vi "ProbeStationAutomation.vi"() -> ()   [LabVIEW 2020]
uses:
  Control 2.ctl
  D:/LabviewDXFViewer/LabviewDXFViewer/bin/Release/LabviewDXFViewer.exe
  LabviewDXFViewer/bin/Release/LabviewDXFViewer.exe
  UIReferences.ctl
  WaferAlignmentType.ctl
  <vilib>/Utility/file.llb/Write Delimited Spreadsheet (DBL).vi
  Keithley 2600 Series/Keithley 2600 Series.lvlib
panel:
  in  "StartOxide":refnum<k24>(container)
  out "WaferAlignment":T1
  out "UiDefinition 3":T2
  in  "PathInfos":T3
  in  "UiDefinition 2":T2
  out "SweepInfo":T4
  out "error out":errorcluster
  out "Position 3":i32[](array[numeric])
  out "Position 2":i32[](array[numeric])
  out "Status":string="Please Load/Select probe site list"
  in  "Chip Orientation":i32(ring) items=["Horizontal", "Vertical"]
  in  "TextEditor":refnum<k24>(container)
  out "WaferTestPoints":string
  out "TestPointsLoaded":bool
  out "dxfFile":string
  out "error out 5":errorcluster
  out "Fit Array":string[][](array[string])
  out "error out 4":errorcluster
  out "error out 3":errorcluster
  out "Fit":dbl[][](array[numeric])
  out "IV Scan Data":dbl[][](array[numeric])
  out "Rotation Misalign":dbl[](array[numeric])
  out "Scale Misalign":dbl
  out "Position 1":i32[](array[numeric])
  in  "Microsites":refnum<k24>(container)
  in  "DXFCanvas":refnum<k24>(container)
  in  "WebCamViewer":refnum<k24>(container)
  in  "IV Curves":T5
  in  "Tab Control":T6(tab)
  in  "ClearPositions":bool
  in  "User":string
  in  "resetcontact":bool
  in  "EnableJoystick":bool
  in  "StartCycle":refnum<k24>(container)
  in  "Version":string
  in  "Experiment":string
  in  "Lower":refnum<k24>(container)
  in  "Raise":refnum<k24>(container)
  in  "West":refnum<k24>(container)
  in  "East":refnum<k24>(container)
  in  "North":refnum<k24>(container)
  in  "South":refnum<k24>(container)
  in  "Align Position 1":bool
  in  "Platten Move":refnum<k24>(container)
  in  "Masks":string(combo)
  in  "Move Position 1":bool
  in  "Align Position 3":bool
  in  "Position 3":bool
  in  "Align Position 2":bool
  in  "Position 2":bool
  in  "Die":string
  in  "Wafer":string
  in  "Jog (um) 2":dbl=100.0
  in  "Jog (um)":dbl=500.0
  in  "Load Mask":bool
  in  "Save Wafer":bool
  in  "Lift Distance (um)":dbl=2000.0
  in  "Quit":bool
  out "In Contact":bool
  out "Motor Position":string
  in  "Save Tag":string
  out "Capacitance":dbl
  in  "Current Range (A)":dbl=1e-10
  in  "Junction":string(combo)="None"
  in  "Sweeps":dbl=2.0
  in  "Number Points":dbl=200.0
  in  "Minimum (mV)":dbl=-100.0
  in  "Maxiumum (mV)":dbl=100.0
  in  "Source Measure Unit Channel (0: Channel A)":i32(ring) items=["Channel A", "Channel B"]
  in  "VISA resource name":refnum<visa-resource-name>="Keithley_2636A"
  in  "Scan":bool
  in  "Save Scan":bool
  out "Conductance":dbl
  out "Intercept":dbl
  out "XY Graph":cluster{"x":timestamp, "y":dbl}[](graph)
  in  "Steps Per micron":dbl=0.629
  in  "Stepper Controller Port":i32=3
  out "GetCameras":string[](array[string])
  in  "Wafer Definition File":path=path "C:/Users/User/Desktop/Automation/ASU FG Mask 21.08.26.dxf"
  in  "Wafer Units to microns":dbl=1.0
  in  "Data Path":path=path "C:/Users/User/Desktop/Automation/data"
  # "Run Oxide"
  # "Optional Tags"
  # "Jog Platten"
  # "Platten Altitude"
  # "Run IVs"
  # "Cycle Step"
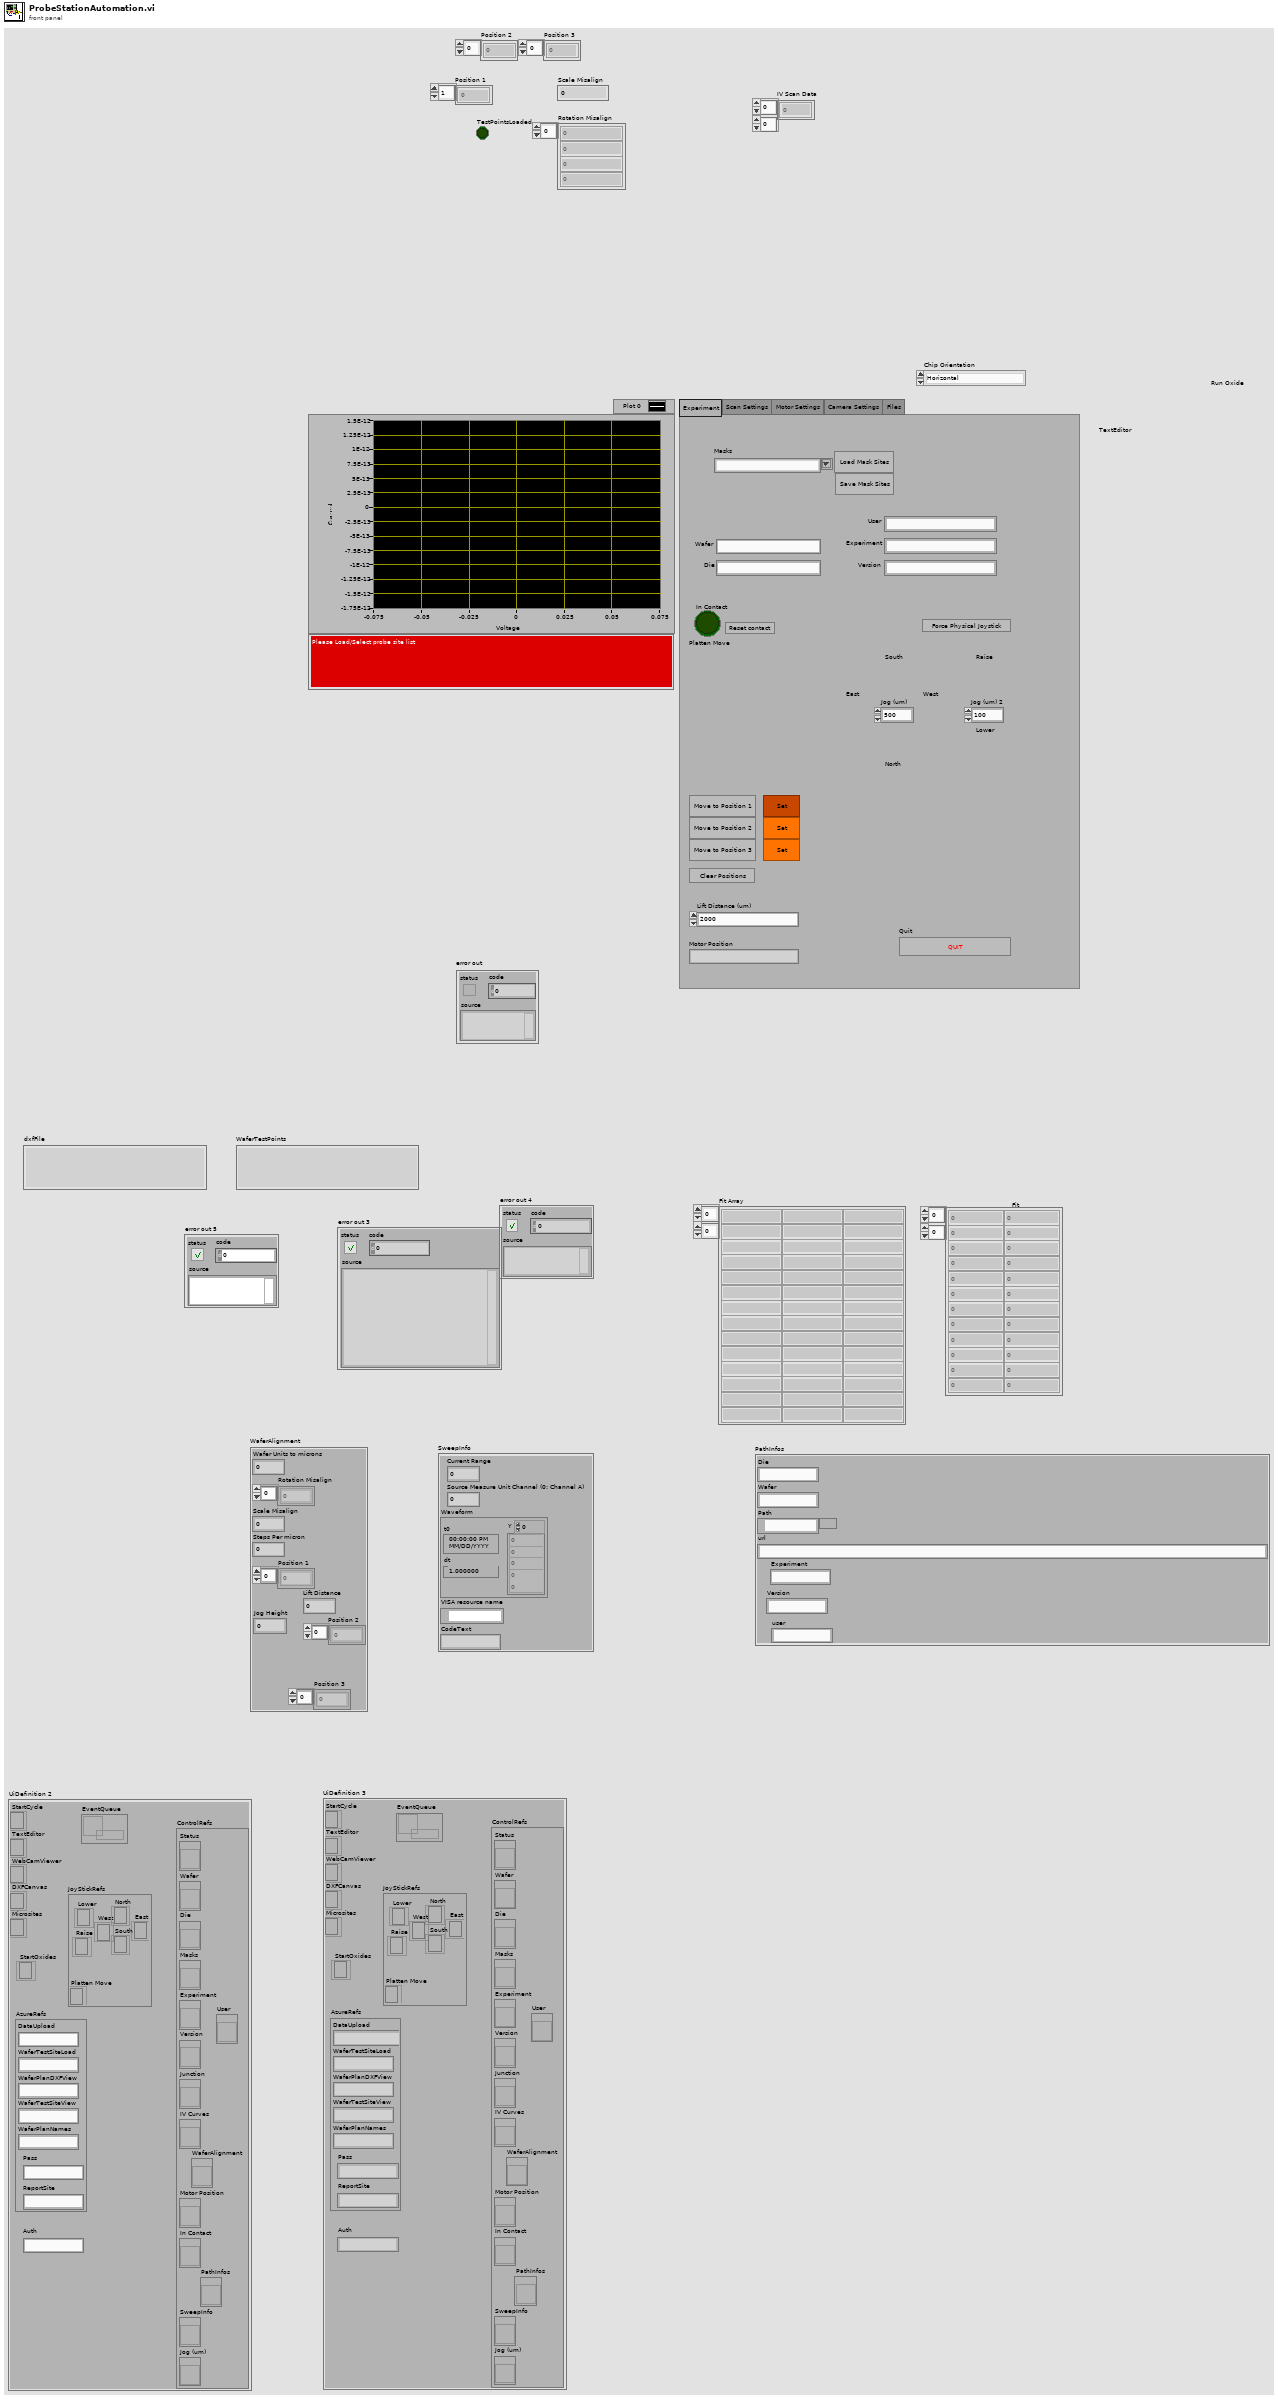
[diagram p1: front panel]
types:
  T1 = typedef "WaferAlignmentType.ctl" = cluster{"Wafer Units to microns":dbl, "Rotation Misalign":dbl[], "Scale Misalign":dbl, "Steps Per micron":dbl, "Position 1":i32[], "Position 2":i32[], "Lift Distance":i32, "Position 3":i32[], "Jog Height":i32}
  T2 = typedef "UIReferences.ctl" = cluster{"StartCycle":refnum<k24>, "TextEditor":refnum<k24>, "WebCamViewer":refnum<k24>, "DXFCanvas":refnum<k24>, "Microsites":refnum<k24>, "JoyStickRefs":cluster{"North":refnum<k24>, "Lower":refnum<k24>, "Raise":refnum<k24>, "Platten Move":refnum<k24>, "West":refnum<k24>, "East":refnum<k24>, "South":refnum<k24>}, "AzureRefs":cluster{"DataUpload":string, "WaferTestSiteLoad":string, "WaferPlanDXFView":string, "WaferTestSiteView":string, "WaferPlanNames":string, "Pass":string, "ReportSite":string}, "ControlRefs":cluster{"Status":refnum<vi>, "Wafer":refnum<vi>, "Die":refnum<vi>, "Masks":refnum<vi>, "Experiment":refnum<vi>, "Version":refnum<vi>, "Junction":refnum<vi>, "IV Curves":refnum<vi>, "Motor Position":refnum<vi>, "In Contact":refnum<vi>, "SweepInfo":refnum<vi>, "Jog (um)":refnum<vi>, "PathInfos":refnum<vi>, "User":refnum<vi>, "WaferAlignment":refnum<vi>}, "EventQueue":refnum<queue>, "StartOxides":refnum<k24>, "Auth":string}
  T3 = cluster{"Die":string, "Wafer":string, "Path":path, "url":string, "Experiment":string, "Version":string, "user":string}
  T4 = cluster{"Current Range":dbl, "Source Measure Unit Channel (0: Channel A)":i32, "Waveform":waveform(dbl), "VISA resource name":refnum<visa-resource-name>, "CodeText":string}
  T5 = typedef "Control 2.ctl" = cluster{"Y":dbl[], "Current (A)":dbl[]}
  T6 = enum32{"Experiment", "Scan Settings", "Motor Settings", "Camera Settings", "Files"}
  T7 = cluster{"DataUpload":string, "WaferTestSiteLoad":string, "WaferPlanDXFView":string, "WaferTestSiteView":string, "WaferPlanNames":string, "Pass":string, "ReportSite":string}
  T8 = cluster{"North":refnum<k24>, "Lower":refnum<k24>, "Raise":refnum<k24>, "Platten Move":refnum<k24>, "West":refnum<k24>, "East":refnum<k24>, "South":refnum<k24>}
  T9 = cluster{"Status":refnum<vi>, "Wafer":refnum<vi>, "Die":refnum<vi>, "Masks":refnum<vi>, "Experiment":refnum<vi>, "Version":refnum<vi>, "Junction":refnum<vi>, "IV Curves":refnum<vi>, "Motor Position":refnum<vi>, "In Contact":refnum<vi>, "SweepInfo":refnum<vi>, "Jog (um)":refnum<vi>, "PathInfos":refnum<vi>, "User":refnum<vi>, "WaferAlignment":refnum<vi>}
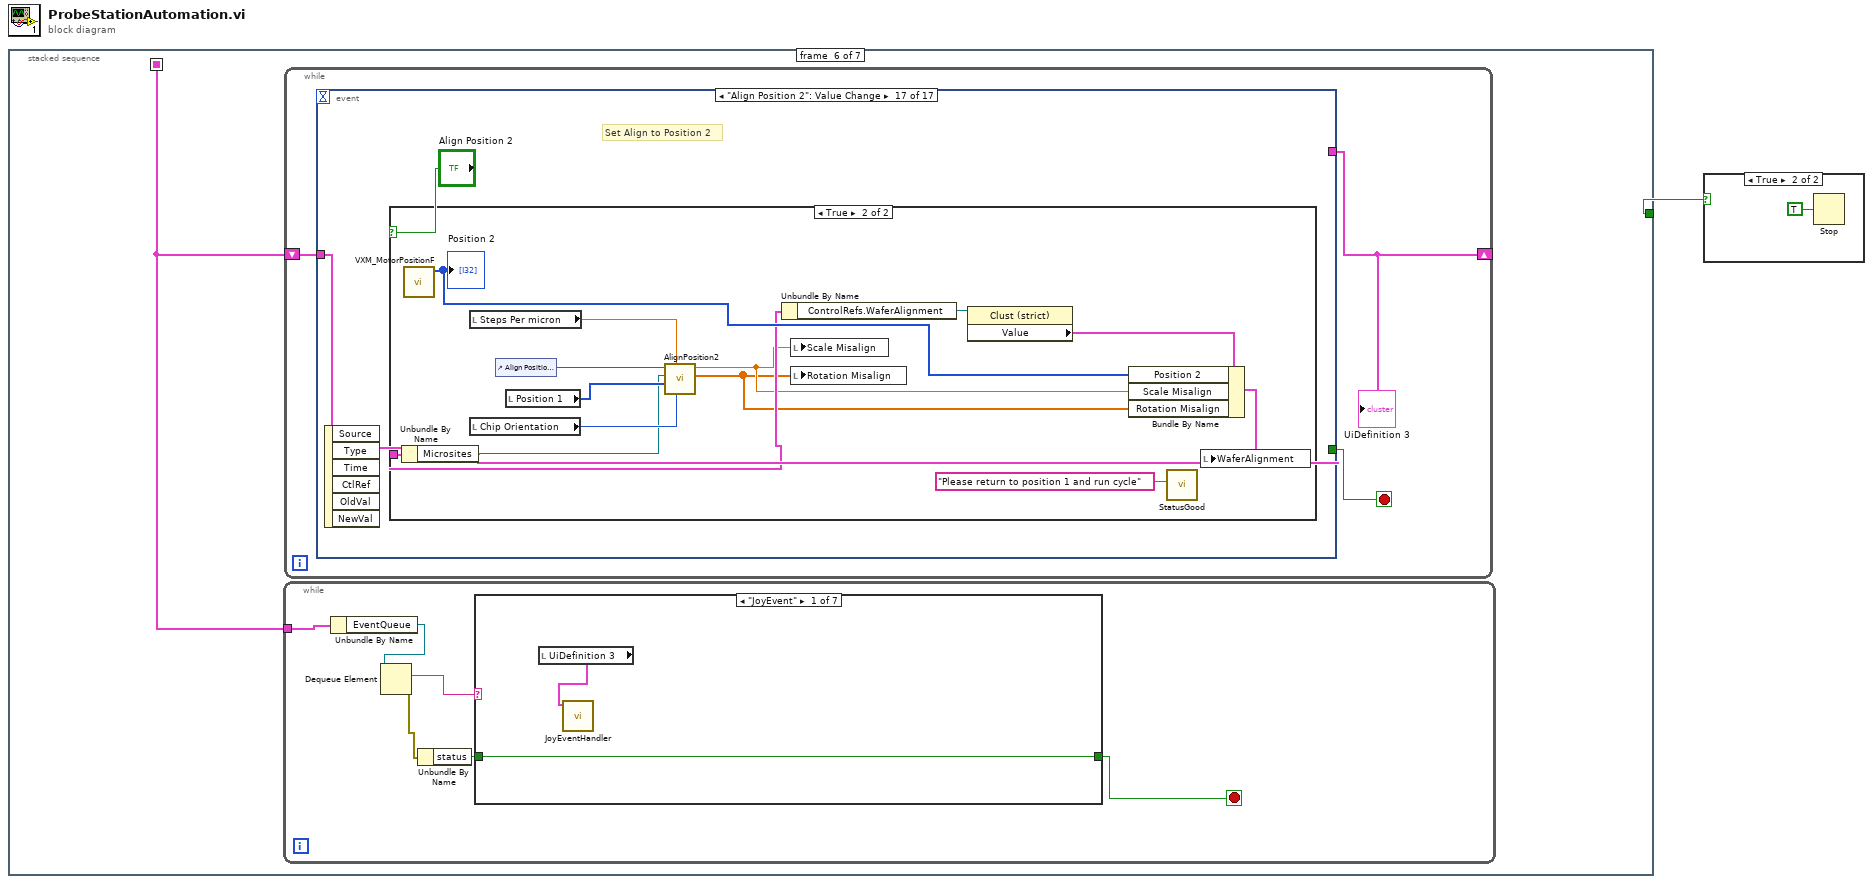
[diagram p0: block diagram]
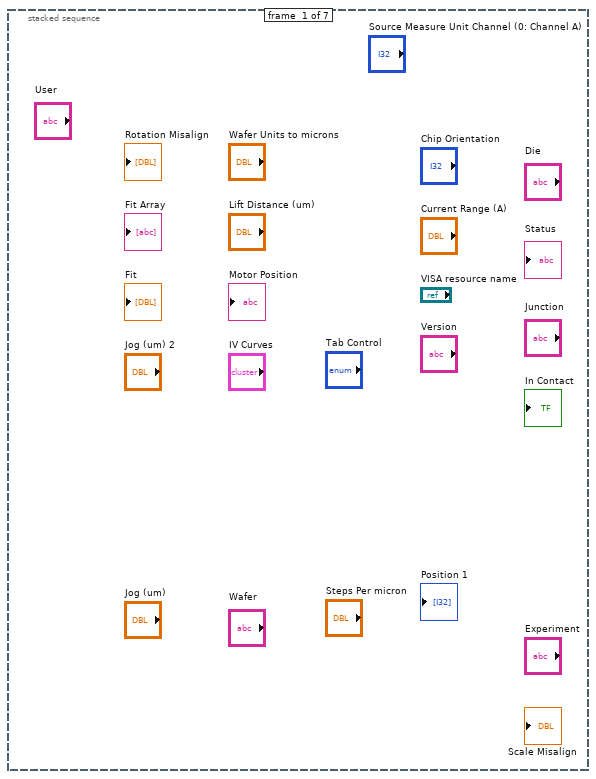
[diagram p3: hidden frame]
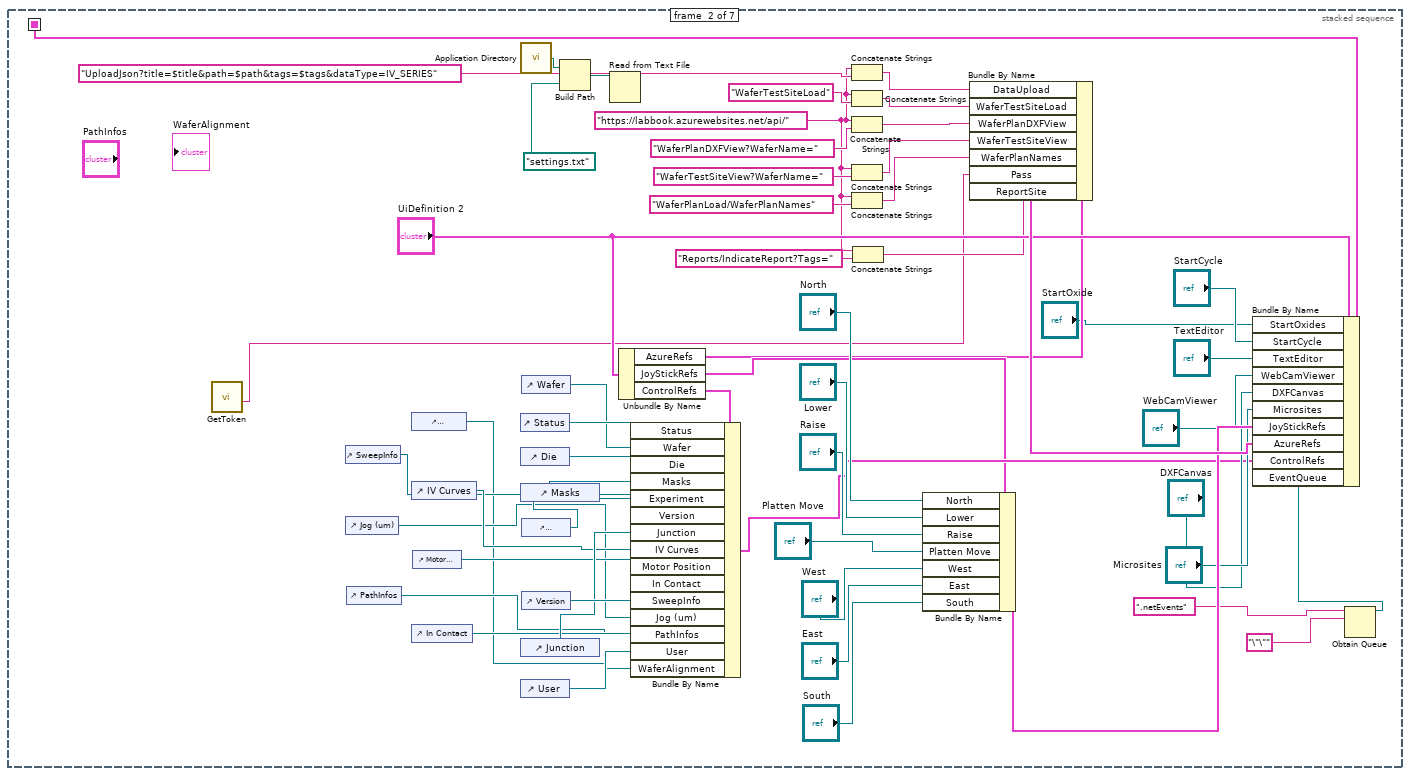
[diagram p4: hidden frame]
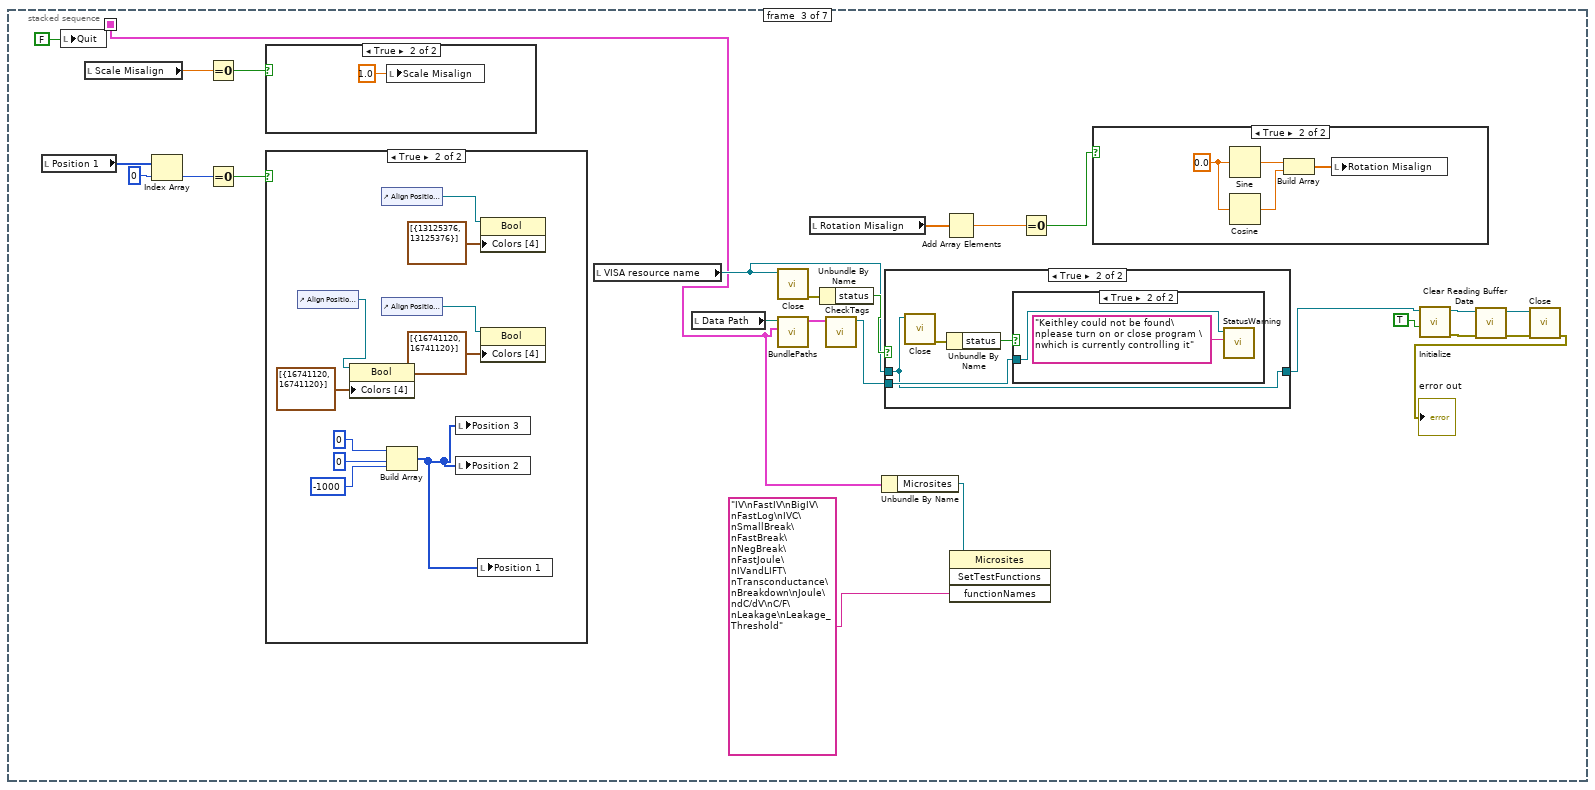
[diagram p5: hidden frame]
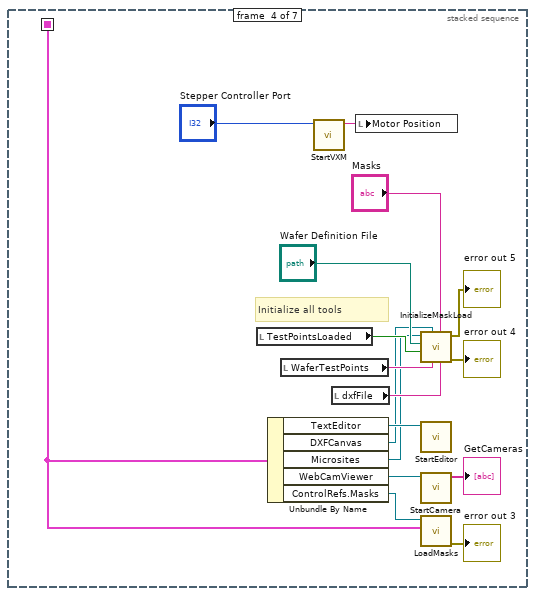
[diagram p11: hidden frame]
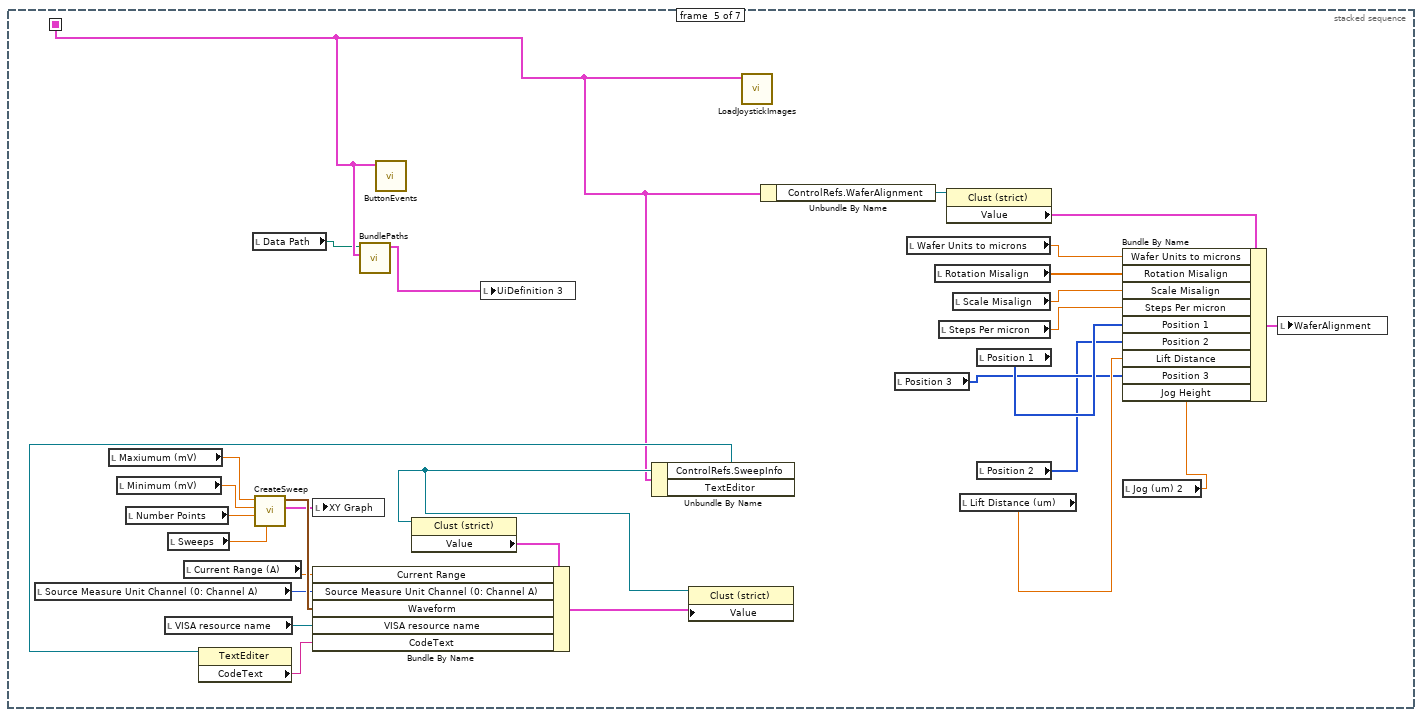
[diagram p12: hidden frame]
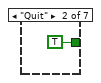
[diagram p13: hidden frame]
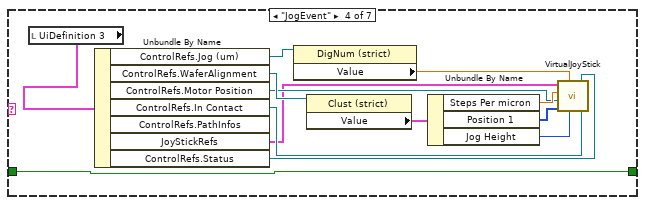
[diagram p15: hidden frame]
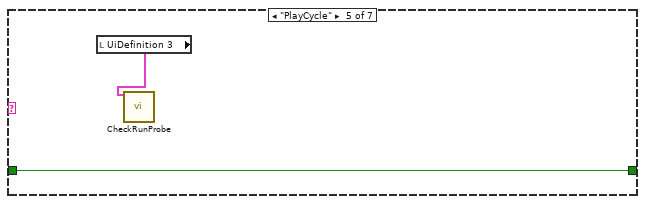
[diagram p16: hidden frame]
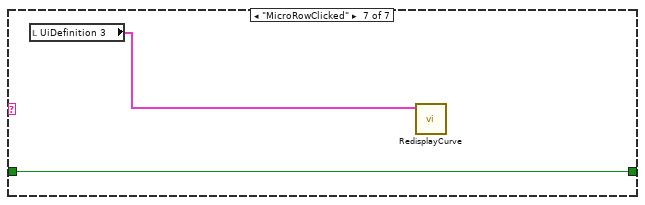
[diagram p18: hidden frame]
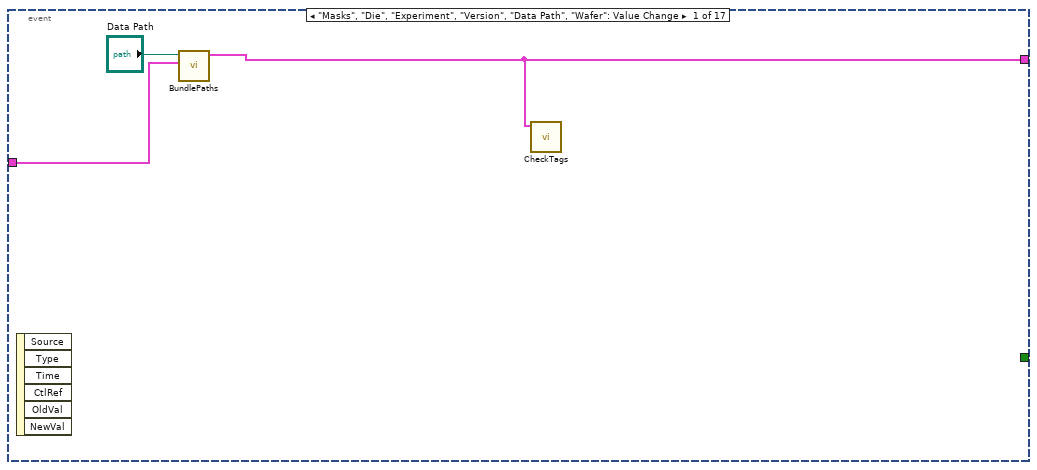
[diagram p19: hidden frame]
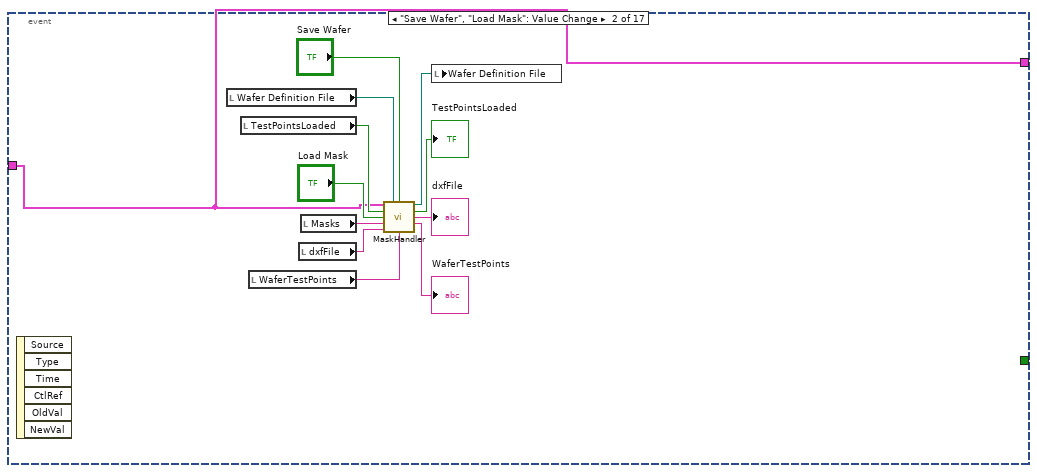
[diagram p20: hidden frame]
diagram:
  n1 = stacked-sequence {
    seq-local: [_ w44 _ _ _ _ _] -> [_ _ w60 w106 w125 w152 _]
    tunnel: [_ _ _ _ _ _ TRUE ("Quit")] -> w1
    frame #0 {
    }
    frame #1 {
      w4 = "https://labbook.azurewebsites.net/api/"
      n2 = call "GetToken.vi"() -> ("value"=w2:string)  [unwired: 10 in, 1 out]
      n3 = control-ref of="SweepInfo"() -> (w29:refnum<vi>)
      n4 = control-ref of="Jog (um)"() -> (w28:refnum<vi>)
      n5 = control-ref of="PathInfos"() -> (w27:refnum<vi>)
      n6 = control-ref of="WaferAlignment"() -> (w6:refnum<vi>)
      n7 = control-ref of="IV Curves"() -> (w32:refnum<vi>)
      n8 = control-ref of="In Contact"() -> (w30:refnum<vi>)
      n9 = control-ref of="Motor Position"() -> (w31:refnum<vi>)
      n10 = call <vilib>:"Application Directory.vi"() -> ("Application Directory"=w8:path)
      n11 = control-ref of="Status"() -> (w39:refnum<vi>)
      n12 = control-ref of="Die"() -> (w37:refnum<vi>)
      n13 = control-ref of="Masks"() -> (w36:refnum<vi>)
      n14 = control-ref of="Junction"() -> (w33:refnum<vi>)
      n15 = control-ref of="User"() -> (w22:refnum<vi>)
      n16 = control-ref of="Wafer"() -> (w38:refnum<vi>)
      n17 = control-ref of="Experiment"() -> (w35:refnum<vi>)
      n18 = control-ref of="Version"() -> (w34:refnum<vi>)
      n19 = Build Path(base path=w8, name or relative path=path "settings.txt" ("file (use dialog)")) -> (appended path=w10:path)
      n20 = Read from Text File(file (use dialog)=w10) -> ()  [unwired: 3 in, 4 out]
      n21 = Unbundle By Name("UiDefinition 2") -> ("AzureRefs"=w21:T7, "JoyStickRefs"=w26:T8, "ControlRefs"=w41:T9)
      n22 = Bundle By Name(cluster=w41, "Status"=w39, "Wafer"=w38, "Die"=w37, "Masks"=w36, "Experiment"=w35, "Version"=w34, "Junction"=w33, "IV Curves"=w32, "Motor Position"=w31, "In Contact"=w30, "SweepInfo"=w29, "Jog (um)"=w28, "PathInfos"=w27, "User"=w22, "WaferAlignment"=w6) -> (w40:T9)
      n23 = Concatenate Strings(w4, "UploadJson?title=$title&path=$path&tags=$tags&dataType=IV_SERIES" ("url")) -> (w20:string)
      n24 = Concatenate Strings(w4, "WaferTestSiteLoad" ("url")) -> (w17:string)
      n25 = Concatenate Strings(w4, "WaferPlanDXFView?WaferName=" ("url")) -> (w15:string)
      n26 = Concatenate Strings(w4, "WaferTestSiteView?WaferName=" ("url")) -> (w13:string)
      n27 = Concatenate Strings(w4, "WaferPlanLoad/WaferPlanNames" ("url")) -> (w11:string)
      n28 = Concatenate Strings(w4, "Reports/IndicateReport?Tags=" ("string")) -> (w5:string)
      n29 = Bundle By Name(cluster=w26, "North"="North", "Lower"="Lower", "Raise"="Raise", "Platten Move"="Platten Move", "West"="West", "East"="East", "South"="South") -> (w53:T8)
      n30 = Bundle By Name(cluster=w21, "DataUpload"=w20, "WaferTestSiteLoad"=w17, "WaferPlanDXFView"=w15, "WaferTestSiteView"=w13, "WaferPlanNames"=w11, "Pass"=w2, "ReportSite"=w5) -> (w57:T7)
      n31 = Obtain Queue(name (unnamed)=".netEvents", element data type="\"\"") -> (queue out=w23:refnum<queue>)  [unwired: 3 in, 2 out]
      n32 = Bundle By Name(cluster="UiDefinition 2", "StartOxides"="StartOxide", "StartCycle"="StartCycle", "TextEditor"="TextEditor", "WebCamViewer"="WebCamViewer", "DXFCanvas"="DXFCanvas", "Microsites"="Microsites", "JoyStickRefs"=w53, "AzureRefs"=w57, "ControlRefs"=w40, "EventQueue"=w23) -> (w44:T2)
    }
    frame #2 {
      n33 = local read "Position 1"() -> (w82:i32[])
      n34 = local write "Quit"(FALSE) -> ()
      n35 = local read "Scale Misalign"() -> (w77:dbl)
      n36 = Index Array(array=w82, index=0) -> (element=w83:i32)
      n37 = Equal To 0?(x=w77) -> (x = 0?=w76:bool)
      n38 = Equal To 0?(x=w83) -> (x = 0?=w81:bool)
      n39 = case shown="True" w76 {
        frame False {
        }
        frame True {
          n40 = local write "Scale Misalign"(1.0 ("Scale Misalign")) -> ()
        }
      }
      n41 = case shown="True" w81 {
        frame False {
        }
        frame True {
          n42 = control-ref of="Align Position 3"() -> (w91:refnum<vi>)
          n43 = property class="Bool"(reference=w91, "Colors [4]"=cluster{u32, u32}[] [{16741120, 16741120}]) -> ()  [unwired: 1 in, 2 out]
          n44 = control-ref of="Align Position 1"() -> (w100:refnum<vi>)
          n45 = control-ref of="Align Position 2"() -> (w98:refnum<vi>)
          n46 = Build Array(0 ("Y"), 0 ("X"), -1000) -> (w93:i32[])
          n47 = local write "Position 3"(w93) -> ()
          n48 = local write "Position 2"(w93) -> ()
          n49 = local write "Position 1"(w93) -> ()
          n50 = property class="Bool"(reference=w100, "Colors [4]"=cluster{u32, u32}[] [{13125376, 13125376}]) -> ()  [unwired: 1 in, 2 out]
          n51 = property class="Bool"(reference=w98, "Colors [4]"=cluster{u32, u32}[] [{16741120, 16741120}]) -> ()  [unwired: 1 in, 2 out]
        }
      }
      n52 = local read "VISA resource name"() -> (w69:refnum<visa-resource-name>)
      n53 = local read "Data Path"() -> (w66:path)
      n54 = call "Close.vi"("VISA resource name"=w69) -> ("error out"=w73:errorcluster)  [unwired: 10 in]
      n55 = call "BundlePaths.vi"("Data Path"=w66, "UiDefinition 2"=w60) -> ("UiDefinition 3"=w67:T2)  [unwired: 8 in]
      n56 = local read "Rotation Misalign"() -> (w80:dbl[])
      n57 = Unbundle By Name(w73) -> ("status"=w72:bool)
      n58 = call "CheckTags.vi"("UiDefinition 2"=w67) -> ("StatusOut"=w71:refnum<vi>)  [unwired: 10 in]
      n59 = Unbundle By Name(w60) -> ("Microsites"=w59:refnum<k24>)
      n60 = case shown="True" w72 {
        tunnel: w71 -> [_ w88]
        tunnel: w69 -> [w84 w87]
        tunnel: [w84 w87] -> w68
        frame False {
        }
        frame True {
          n61 = call "Close.vi"("VISA resource name"=w87) -> ("error out"=w86:errorcluster)  [unwired: 10 in]
          n62 = Unbundle By Name(w86) -> ("status"=w85:bool)
          n63 = case shown="True" w85 {
            tunnel: w88 -> [_ w89]
            frame False {
            }
            frame True {
              n64 = call "StatusWarning.vi"("Text.Text"="Keithley could not be found\nplease turn on or close program \nwhich is currently controlling it", "String in"=w89) -> ()  [unwired: 10 in]
            }
          }
        }
      }
      n65 = Add Array Elements(numeric array=w80) -> (sum=w79:dbl)
      n66 = invoke class="Microsites" method="SetTestFunctions"(reference=w59, "functionNames"="IV\nFastIV\nBigIV\nFastLog\nIVC\nSmallBreak\nFastBreak\nNegBreak\nFastJoule\nIVandLIFT\nTransconductance\nBreakdown\nJoule\ndC/dV\nC/F\nLeakage\nLeakage_Threshold") -> ()  [unwired: 2 in, 4 out]
      n67 = Equal To 0?(x=w79) -> (x = 0?=w78:bool)
      n68 = case shown="True" w78 {
        frame False {
        }
        frame True {
          w101 = 0.0 ("x")
          n69 = Sine(x=w101) -> (sin(x)=w104:dbl)
          n70 = Cosine(x=w101) -> (cos(x)=w103:dbl)
          n71 = Build Array(w104, w103) -> (w102:dbl[])
          n72 = local write "Rotation Misalign"(w102) -> ()
        }
      }
      n73 = call "Initialize.vi"("Reset (True)"=TRUE, "VISA resource name"=w68) -> ("error out"=w64:errorcluster, "VISA resource name out"=w65:refnum<visa-resource-name>)  [unwired: 8 in]
      n74 = call "Clear Reading Buffer Data.vi"("error in (no error)"=w64, "VISA resource name"=w65) -> ("error out"=w63:errorcluster, "VISA resource name out"=w62:refnum<visa-resource-name>)  [unwired: 8 in]
      n75 = call "Close.vi"("error in (no error)"=w63, "VISA resource name"=w62) -> ("error out"=→"error out":errorcluster)  [unwired: 9 in]
    }
    frame #3 {
      # "Initialize all tools"
      n76 = local read "TestPointsLoaded"() -> (w117:bool)
      n77 = Unbundle By Name(w106) -> ("TextEditor"=w111:refnum<k24>, "DXFCanvas"=w110:refnum<k24>, "Microsites"=w109:refnum<k24>, "WebCamViewer"=w108:refnum<k24>, "ControlRefs.Masks"=w107:refnum<vi>)
      n78 = local read "WaferTestPoints"() -> (w116:string)
      n79 = call "StartVXM.vi"("Stepper Controller Port"="Stepper Controller Port") -> ("String"=w112:string)  [unwired: 10 in]
      n80 = local read "dxfFile"() -> (w115:string)
      n81 = local write "Motor Position"(w112) -> ()
      n82 = call "InitializeMaskLoad.vi"("dxfFile"=w115, "Masks"="Masks", "WaferTestPoints"=w116, "DXFCanvas"=w110, "TestPointsLoaded"=w117, "Wafer Definition File"="Wafer Definition File", "MicrositesRef"=w109) -> ("error out"=→"error out 4":errorcluster, "error out 5"=→"error out 5":errorcluster)  [unwired: 3 in]
      n83 = call "StartEditor.vi"("CodeEditorRef"=w111) -> ()  [unwired: 11 in]
      n84 = call "StartCamera.vi"("WebCamViewerRef"=w108) -> ("GetCameras"=→"GetCameras":string[])  [unwired: 10 in]
      n85 = call "LoadMasks.vi"("UiDefinition 2"=w106, "ComboBox in"=w107) -> ("error out"=→"error out 3":errorcluster)  [unwired: 9 in]
    }
    frame #4 {
      n86 = local read "Source Measure Unit Channel (0: Channel A)"() -> (w134:i32)
      n87 = local read "Maxiumum (mV)"() -> (w131:dbl)
      n88 = local read "Minimum (mV)"() -> (w130:dbl)
      n89 = local read "Number Points"() -> (w129:dbl)
      n90 = local read "VISA resource name"() -> (w139:refnum<visa-resource-name>)
      n91 = local read "Sweeps"() -> (w128:dbl)
      n92 = local read "Current Range (A)"() -> (w133:dbl)
      n93 = local read "Data Path"() -> (w123:path)
      n94 = call "CreateSweep.vi"("Sweeps"=w128, "Number Points"=w129, "Minimum Voltage"=w130, "Maxiumum Voltage"=w131) -> ("XY pairs"=w127:cluster{"x":timestamp, "y":dbl}[], "Waveform"=w135:waveform(dbl))  [unwired: 6 in]
      n95 = local write "XY Graph"(w127) -> ()
      n96 = call "BundlePaths.vi"("Data Path"=w123, "UiDefinition 2"=w125) -> ("UiDefinition 3"=w124:T2)  [unwired: 8 in]
      n97 = call "ButtonEvents.vi"("UiDefinition"=w125) -> ()  [unwired: 11 in]
      n98 = local write "UiDefinition 3"(w124) -> ()
      n99 = Unbundle By Name(w125) -> ("ControlRefs.SweepInfo"=w137:refnum<vi>, "TextEditor"=w138:refnum<k24>)
      n100 = property class="TextEditer"(reference=w138) -> ("CodeText"=w140:string)  [unwired: 1 in, 2 out]
      n101 = property class="Clust (strict)"(reference=w137) -> ("Value"=w136:T4)  [unwired: 1 in, 2 out]
      n102 = Bundle By Name(cluster=w136, "Current Range"=w133, "Source Measure Unit Channel (0: Channel A)"=w134, "Waveform"=w135, "VISA resource name"=w139, "CodeText"=w140) -> (w132:T4)
      n103 = property class="Clust (strict)"(reference=w137, "Value"=w132) -> ()  [unwired: 1 in, 2 out]
      n104 = call "LoadJoystickImages.vi"("UiDefinition 2"=w125) -> ()  [unwired: 11 in]
      n105 = Unbundle By Name(w125) -> ("ControlRefs.WaferAlignment"=w151:refnum<vi>)
      n106 = local read "Position 3"() -> (w143:i32[])
      n107 = local read "Wafer Units to microns"() -> (w148:dbl)
      n108 = local read "Rotation Misalign"() -> (w147:dbl[])
      n109 = local read "Steps Per micron"() -> (w141:dbl)
      n110 = property class="Clust (strict)"(reference=w151) -> ("Value"=w150:T1)  [unwired: 1 in, 2 out]
      n111 = local read "Scale Misalign"() -> (w146:dbl)
      n112 = local read "Lift Distance (um)"() -> (w144:dbl)
      n113 = local read "Position 1"() -> (w145:i32[])
      n114 = local read "Position 2"() -> (w142:i32[])
      n115 = local read "Jog (um) 2"() -> (w126:dbl)
      n116 = Bundle By Name(cluster=w150, "Wafer Units to microns"=w148, "Rotation Misalign"=w147, "Scale Misalign"=w146, "Steps Per micron"=w141, "Position 1"=w145, "Position 2"=w142, "Lift Distance"=w144, "Position 3"=w143, "Jog Height"=w126) -> (w149:T1)
      n117 = local write "WaferAlignment"(w149) -> ()
    }
    frame #5 {
      n118 = while {
        tunnel: w152 -> [w153]
        stop <- w154 stop-if-true
        n119 = Unbundle By Name(w153) -> ("EventQueue"=w157:refnum<queue>)
        n120 = Dequeue Element(queue=w157) -> (element=w158:string, error out=w156:errorcluster)  [unwired: 2 in, 2 out]
        n121 = Unbundle By Name(w156) -> ("status"=w155:bool)
        n122 = case shown="\"JoyEvent\"" w158 {
          tunnel: w155 -> [w160 _ w162 w164 w177 w178 w180]
          tunnel: [w160 TRUE ("status") w162 w164 w177 w178 w180] -> w154
          frame "JoyEvent" {
            n123 = local read "UiDefinition 3"() -> (w159:T2)
            n124 = call "JoyEventHandler.vi"("UiDefinition"=w159) -> ()  [unwired: 11 in]
          }
          frame "Quit" {
          }
          frame Default {
          }
          frame "JogEvent" {
            n125 = local read "UiDefinition 3"() -> (w163:T2)
            n126 = Unbundle By Name(w163) -> ("ControlRefs.Jog (um)"=w167:refnum<vi>, "ControlRefs.WaferAlignment"=w175:refnum<vi>, "ControlRefs.Motor Position"=w172:refnum<vi>, "ControlRefs.In Contact"=w170:refnum<vi>, "JoyStickRefs"=w168:T8, "ControlRefs.Status"=w165:refnum<vi>)  [unwired: 1 out]
            n127 = property class="DigNum (strict)"(reference=w167) -> ("Value"=w166:dbl)  [unwired: 1 in, 2 out]
            n128 = property class="Clust (strict)"(reference=w175) -> ("Value"=w174:T1)  [unwired: 1 in, 2 out]
            n129 = Unbundle By Name(w174) -> ("Steps Per micron"=w173:dbl, "Position 1"=w171:i32[], "Jog Height"=w169:i32)
            n130 = call "VirtualJoyStick.vi"("In Contact"=w170, "Status"=w165, "Jog (um) raise"=w169, "Jog (um)"=w166, "Position 1"=w171, "Motor Zero"=w172, "Steps Per micron"=w173, "JoyStickRefs"=w168) -> ()
          }
          frame "PlayCycle" {
            n131 = local read "UiDefinition 3"() -> (w176:T2)
            n132 = call "CheckRunProbe.vi"("UiDefinition"=w176) -> ()  [unwired: 15 in]
          }
          frame "OxideCycle" {
          }
          frame "MicroRowClicked" {
            n133 = local read "UiDefinition 3"() -> (w179:T2)
            n134 = call "RedisplayCurve.vi"("UiDefinition 3"=w179) -> ()  [unwired: 11 in]
          }
        }
      }
      n135 = while {
        shift-right: [w182] -> _
        shift-left: w152 -> [w183]
        stop <- w181 stop-if-true
        n136 = event shown="[16] \"Align Position 2\": Value Change" {
          selector: _ -> [_ _ _ _ _ _ _ _ _ _ _ _ _ _ _ _ _]
          dyn-events: _ -> [_ _ _ _ _ _ _ _ _ _ _ _ _ _ _ _ _]
          timeout: _ -> [_ _ _ _ _ _ _ _ _ _ _ _ _ _ _ _ _]
          tunnel: w183 -> [w185 w187 w199 w206 w223 w229 w238 w247 w255 w259 w263 w327 w329 w345 w349 w359 w371]
          tunnel: [w184 w187 w199 w206 w223 w229 w238 w247 w255 w259 w263 w327 w329 w345 w349 w359 w371] -> w182
          tunnel: [_ _ _ _ _ _ "Quit" _ _ _ _ _ _ _ _ _ _] -> w181
          event "Masks", "Die", "Experiment", "Version", "Data Path", "Wafer": Value Change {
            n137 = event-data() -> ()  [unwired: 1 in, 6 out]
            n138 = call "BundlePaths.vi"("Data Path"="Data Path", "UiDefinition 2"=w185) -> ("UiDefinition 3"=w184:T2)  [unwired: 8 in]
            n139 = call "CheckTags.vi"("UiDefinition 2"=w184) -> ()  [unwired: 10 in, 1 out]
          }
          event "Save Wafer", "Load Mask": Value Change {
            n140 = event-data() -> ()  [unwired: 1 in, 6 out]
            n141 = local read "Wafer Definition File"() -> (w195:path)
            n142 = local read "TestPointsLoaded"() -> (w192:bool)
            n143 = local read "WaferTestPoints"() -> (w196:string)
            n144 = local read "dxfFile"() -> (w198:string)
            n145 = local read "Masks"() -> (w189:string)
            n146 = call "MaskHandler.vi"("UiDefinition 2"=w187, "Wafer Definition File"=w195, "Save Wafer"="Save Wafer", "TestPointsLoaded in"=w192, "Load Mask"="Load Mask", "Masks"=w189, "dxfFile"=w198, "WaferTestPoints"=w196) -> ("Path"=w193:path, "TestPointsLoaded out"=→"TestPointsLoaded":bool, "body 2"=→"dxfFile":string, "body"=→"WaferTestPoints":string)  [unwired: 4 in]
            n147 = local write "Wafer Definition File"(w193) -> ()
          }
          event "Scan": Value Change {
            # "On request IV curve"
            n148 = event-data() -> ()  [unwired: 1 in, 6 out]
            n149 = case shown="True" "Scan" {
              tunnel: w199 -> [_ w202]
              frame False {
              }
              frame True {
                n150 = call "SingleIV.vi"("UiDefinition 2"=w202) -> ("appended array"=→"IV Scan Data":dbl[][], "CapacitanceIV"=→"Capacitance":dbl, "slope"=→"Conductance":dbl, "intercept"=→"Intercept":dbl)  [unwired: 11 in]
              }
            }
          }
          event "Align Position 1": Value Change {
            n151 = event-data() -> ()  [unwired: 1 in, 6 out]
            n152 = Unbundle By Name(w206) -> ("ControlRefs.Status"=w207:refnum<vi>)
            n153 = case shown="True" "Align Position 1" {
              tunnel: w207 -> [_ w215]
              tunnel: w206 -> [_ w210]
              frame False {
              }
              frame True {
                n154 = Unbundle By Name(w210) -> ("ControlRefs.WaferAlignment"=w213:refnum<vi>)
                n155 = local write "In Contact"(TRUE) -> ()
                n156 = property class="Clust (strict)"(reference=w213) -> ("Value"=w212:T1)  [unwired: 1 in, 2 out]
                n157 = control-ref of="Align Position 1"() -> (w218:refnum<vi>)
                n158 = call "VXM_MotorPositionF.vi"() -> ("Position"=w211:i32[])  [unwired: 11 in]
                n159 = Bundle By Name(cluster=w212, "Position 1"=w211) -> (w209:T1)
                n160 = local write "Position 1"(w211) -> ()
                n161 = property class="Bool"(reference=w218, "Colors [4]"=cluster{u32, u32}[] [{13816530, 13816530}]) -> ()  [unwired: 1 in, 2 out]
                n162 = local write "WaferAlignment"(w209) -> ()
                n163 = call "StatusGood.vi"("Text.Text"="Align Position 2 or run cycle" ("Status"), "String in"=w215) -> ()  [unwired: 10 in]
              }
            }
          }
          event "Minimum (mV)", "Maxiumum (mV)", "Number Points", "Sweeps": Value Change {
            n164 = event-data() -> ()  [unwired: 1 in, 6 out]
            n165 = Unbundle By Name(w223) -> ("ControlRefs.SweepInfo"=w219:refnum<vi>)
            n166 = call "CreateSweep.vi"("Sweeps"="Sweeps", "Number Points"="Number Points", "Minimum Voltage"="Minimum (mV)", "Maxiumum Voltage"="Maxiumum (mV)") -> ("XY pairs"=→"XY Graph":cluster{"x":timestamp, "y":dbl}[], "Waveform"=w221:waveform(dbl))  [unwired: 6 in]
            n167 = property class="Clust (strict)"(reference=w219) -> ("Value"=w222:T4)  [unwired: 1 in, 2 out]
            n168 = Bundle By Name(cluster=w222, "Waveform"=w221) -> (w220:T4)
            n169 = property class="Clust (strict)"(reference=w219, "Value"=w220) -> ()  [unwired: 1 in, 2 out]
          }
          event "Current Range (A)", "VISA resource name", "Source Measure Unit Channel (0: Channel A)": Value Change {
            n170 = event-data() -> ()  [unwired: 1 in, 6 out]
            n171 = Unbundle By Name(w229) -> ("ControlRefs.SweepInfo"=w232:refnum<vi>, "TextEditor"=w233:refnum<k24>)
            n172 = local read "Source Measure Unit Channel (0: Channel A)"() -> (w234:i32)
            n173 = local read "VISA resource name"() -> (w235:refnum<visa-resource-name>)
            n174 = local read "Current Range (A)"() -> (w236:dbl)
            n175 = property class="Clust (strict)"(reference=w232) -> ("Value"=w230:T4)  [unwired: 1 in, 2 out]
            n176 = property class="TextEditer"(reference=w233) -> ("CodeText"=w237:string)  [unwired: 1 in, 2 out]
            n177 = Bundle By Name(cluster=w230, "Current Range"=w236, "Source Measure Unit Channel (0: Channel A)"=w234, "VISA resource name"=w235, "CodeText"=w237) -> (→"SweepInfo":T4)
          }
          event "Quit": Value Change {
            n178 = event-data() -> ()  [unwired: 1 in, 6 out]
            n179 = Unbundle By Name(w238) -> ("EventQueue"=w240:refnum<queue>)
            n180 = Enqueue Element(queue=w240, element="Quit") -> ()  [unwired: 2 in, 3 out]
          }
          event "Position 1", "Wafer Units to microns", "Rotation Misalign", "Scale Misalign", "Steps Per micron", "Lift Distance (um)", "Jog (um) 2": Value Change {
            n181 = event-data() -> ()  [unwired: 1 in, 6 out]
            n182 = Unbundle By Name(w247) -> ("ControlRefs.WaferAlignment"=w249:refnum<vi>)
            n183 = property class="Clust (strict)"(reference=w249) -> ("Value"=w248:T1)  [unwired: 1 in, 2 out]
            n184 = local read "Wafer Units to microns"() -> (w253:dbl)
            n185 = local read "Rotation Misalign"() -> (w250:dbl[])
            n186 = local read "Lift Distance (um)"() -> (w244:dbl)
            n187 = local read "Steps Per micron"() -> (w251:dbl)
            n188 = local read "Scale Misalign"() -> (w252:dbl)
            n189 = local read "Jog (um) 2"() -> (w243:dbl)
            n190 = local read "Position 1"() -> (w254:i32[])
            n191 = local read "Position 2"() -> (w246:i32[])
            n192 = local read "Position 3"() -> (w245:i32[])
            n193 = Bundle By Name(cluster=w248, "Wafer Units to microns"=w253, "Rotation Misalign"=w250, "Scale Misalign"=w252, "Steps Per micron"=w251, "Position 1"=w254, "Position 2"=w246, "Lift Distance"=w244, "Position 3"=w245, "Jog Height"=w243) -> (w242:T1)
            n194 = local write "WaferAlignment"(w242) -> ()
          }
          event "Move Position 1": Value Change {
            n195 = event-data() -> ()  [unwired: 1 in, 6 out]
            n196 = local read "In Contact"() -> (w258:bool)
            n197 = call "MovePos1.vi"("In Contact in"=w258, "Move Position 1"="Move Position 1", "UiDefinition 2"=w255) -> ("In Contact out"=w257:bool)  [unwired: 8 in]
            n198 = local write "In Contact"(w257) -> ()
          }
          event "Position 2": Value Change {
            n199 = event-data() -> ()  [unwired: 1 in, 6 out]
            n200 = local read "In Contact"() -> (w262:bool)
            n201 = call "MoveToPosition2.vi"("In Contact in"=w262, "Position in"="Position 2", "UiDefinition 2"=w259) -> ("In Contact out"=w261:bool)  [unwired: 8 in]
            n202 = local write "In Contact"(w261) -> ()
          }
          event "Save Scan": Value Change {
            n203 = event-data() -> ()  [unwired: 1 in, 6 out]
            n204 = case shown="True" "Save Scan" {
              tunnel: w263 -> [_ w271]
              frame False {
              }
              frame True {
                n205 = Unbundle By Name(w271) -> ("ControlRefs.PathInfos"=w274:refnum<vi>)  [unwired: 1 out]
                n206 = local read "Junction"() -> (w268:string)
                n207 = property class="Clust (strict)"(reference=w274) -> ("Value"=w273:T3)  [unwired: 1 in, 2 out]
                n208 = Not Equal?(x="None", y=w268) -> (x != y?=w270:bool)
                n209 = local read "IV Scan Data"() -> (w277:dbl[][])
                n210 = Unbundle By Name(w273) -> ("Path"=w266:path, "url"=w272:string)
                n211 = call <vilib>:"Check if File or Folder Exists.vi"("path"=w266) -> ("file or folder exists?"=w267:bool)  [unwired: 8 in, 2 out]
                n212 = case shown="False" w267 {
                  tunnel: w266 -> [w279 w280]
                  tunnel: [w278 w280] -> w265
                  frame False {
                    n213 = Create Folder(path (use dialog)=w279) -> (created path=w278:path)  [unwired: 2 in, 2 out]
                  }
                  frame True {
                  }
                }
                n214 = case shown="True" TRUE {
                  tunnel: w277 -> [_ w289]
                  tunnel: "Save Tag" -> [_ w283]
                  tunnel: w270 -> [_ w285]
                  tunnel: w268 -> [_ w282]
                  tunnel: w265 -> [_ w281]
                  frame False {
                  }
                  frame True {
                    n215 = Empty String/Path?(string/path=w283) -> (empty?=w284:bool)
                    n216 = case shown="True" w285 {
                      tunnel: [w293 FALSE ("cancelled")] -> w288
                      tunnel: [w292 w294] -> w287
                      tunnel: [w291 errorcluster {"status"=FALSE, "code"=0, "source"=""} ("error out")] -> w286
                      tunnel: w284 -> [_ w298]
                      tunnel: w281 -> [w290 w297]
                      tunnel: w283 -> [_ w296]
                      tunnel: w282 -> [_ w295]
                      frame False {
                        n217 = call "File Dialog"("start path"=w290) -> ("selected path"=w292:path, "cancelled"=w293:bool, "error out"=w291:errorcluster)  [unwired: 11 in, 1 out]
                      }
                      frame True {
                        n218 = case shown="True" w298 {
                          tunnel: w297 -> [w307 w311]
                          tunnel: [w306 w312] -> w294
                          tunnel: w296 -> [w302 _]
                          tunnel: w295 -> [w304 w310]
                          frame False {
                            n219 = Concatenate Strings(w304, "_" ("string"), w302, ".csv" ("string")) -> (w305:string)
                            n220 = Build Path(base path=w307, name or relative path=w305) -> (appended path=w306:path)
                          }
                          frame True {
                            n221 = Concatenate Strings(w310, "_m.csv" ("string")) -> (w309:string)
                            n222 = Build Path(base path=w311, name or relative path=w309) -> (appended path=w312:path)
                          }
                        }
                      }
                    }
                    n223 = case shown="False" w288 {
                      tunnel: w289 -> [w314 _]
                      tunnel: w287 -> [w313 _]
                      tunnel: w286 -> [_ _]
                      frame False {
                        n224 = call-poly <vilib>:"Write Delimited Spreadsheet.vi"("file path (dialog if empty)"=w313, "format (%.3f)"="%.9e", "2D data"=w314, "transpose? (no:F)"=TRUE, "delimiter (\\t)"="," ("delimiter (\\t)")) -> ()  [unwired: 9 in, 2 out]
                      }
                      frame True {
                      }
                    }
                  }
                }
                n225 = case shown="True" w270 {
                  tunnel: w277 -> [_ w326]
                  tunnel: w272 -> [_ w324]
                  tunnel: w268 -> [_ w323]
                  tunnel: w271 -> [_ w321]
                  tunnel: "Save Tag" -> [_ w319]
                  frame False {
                  }
                  frame True {
                    n226 = Concatenate Strings(w319, "|" ("string"), w323) -> (w320:string)
                    n227 = Search and Replace String(input string=w324, search string="JuncName" ("string"), replace string=w320) -> (result string=w325:string)  [unwired: 5 in, 3 out]
                    n228 = call "UploadIV.vi"("UiDefinition 2"=w321, "IV Scan Data"=w326, "url"=w325) -> ()  [unwired: 9 in]
                  }
                }
              }
            }
          }
          event "EnableJoystick": Value Change {
            n229 = event-data() -> ()  [unwired: 1 in, 6 out]
            n230 = case shown="True" "EnableJoystick" {
              frame False {
              }
              frame True {
                n231 = call "ReturnToJoystick.vi"() -> ()  [unwired: 12 in]
              }
            }
          }
          event "resetcontact": Value Change {
            n232 = event-data() -> ()  [unwired: 1 in, 6 out]
            n233 = case shown="True" "resetcontact" {
              tunnel: w329 -> [_ w334]
              frame False {
              }
              frame True {
                n234 = call "VXM_MotorPositionF.vi"() -> ("Position"=w343:i32[])  [unwired: 11 in]
                n235 = local write "In Contact"(FALSE ("In Contact")) -> ()
                n236 = Index Array(array=w343, index=2) -> (element=w341:i32)
                n237 = Add(x=-3000, y=w341) -> (x+y=w338:i32)
                n238 = call "StatusGood.vi"("Text.Text"="Please reset position 1") -> ()  [unwired: 11 in]
                n239 = Unbundle By Name(w334) -> ("ControlRefs.WaferAlignment"=w335:refnum<vi>)
                n240 = local read "Position 1"() -> (w339:i32[])
                n241 = property class="Clust (strict)"(reference=w335) -> ("Value"=w333:T1)  [unwired: 1 in, 2 out]
                n242 = Replace Array Subset(array=w339, new element=w338, index=2) -> (w332:i32[])
                n243 = local write "Position 1"(w332) -> ()
                n244 = Bundle By Name(cluster=w333, "Position 1"=w332) -> (w331:T1)
                n245 = local write "WaferAlignment"(w331) -> ()
              }
            }
          }
          event "Position 3": Value Change {
            # "Move to position 3"
            n246 = event-data() -> ()  [unwired: 1 in, 6 out]
            n247 = local read "In Contact"() -> (w348:bool)
            n248 = call "MovePos3.vi"("In Contact in"=w348, "Position 3"="Position 3", "UiDefinition 2"=w345) -> ("In Contact out"=w347:bool)  [unwired: 8 in]
            n249 = local write "In Contact"(w347) -> ()
          }
          event "Align Position 3": Value Change {
            n250 = event-data() -> ()  [unwired: 1 in, 6 out]
            n251 = case shown="True" "Align Position 3" {
              tunnel: w349 -> [_ w353]
              frame False {
              }
              frame True {
                n252 = call "VXM_MotorPositionF.vi"() -> ("Position"=w351:i32[])  [unwired: 11 in]
                "Position 3" <- w351
                n253 = control-ref of="Align Position 3"() -> (w357:refnum<vi>)
                n254 = property class="Bool"(reference=w357, "Colors [4]"=cluster{u32, u32}[] [{13816530, 13816530}]) -> ()  [unwired: 1 in, 2 out]
                n255 = Unbundle By Name(w353) -> ("ControlRefs.WaferAlignment"=w355:refnum<vi>)
                n256 = property class="Clust (strict)"(reference=w355) -> ("Value"=w354:T1)  [unwired: 1 in, 2 out]
                n257 = Bundle By Name(cluster=w354, "Position 3"=w351) -> (w352:T1)
                n258 = local write "WaferAlignment"(w352) -> ()
                n259 = call "StatusGood.vi"("Text.Text"="Please return to position 1 and run cycle" ("Status")) -> ()  [unwired: 11 in]
              }
            }
          }
          event "ClearPositions": Value Change {
            n260 = event-data() -> ()  [unwired: 1 in, 6 out]
            n261 = case shown="True" "ClearPositions" {
              tunnel: w359 -> [_ w366]
              frame False {
              }
              frame True {
                w362 = cluster{u32, u32}[] [{16741120, 16741120}] ("Colors [4]")
                w361 = i32[] [] ("Position 3")
                n262 = control-ref of="Align Position 1"() -> (w363:refnum<vi>)
                n263 = control-ref of="Align Position 3"() -> (w367:refnum<vi>)
                n264 = property class="Bool"(reference=w367, "Colors [4]"=w362) -> ()  [unwired: 1 in, 2 out]
                n265 = control-ref of="Align Position 2"() -> (w364:refnum<vi>)
                n266 = Unbundle By Name(w366) -> ("ControlRefs.WaferAlignment"=w365:refnum<vi>)
                n267 = property class="Bool"(reference=w364, "Colors [4]"=w362) -> ()  [unwired: 1 in, 2 out]
                n268 = property class="Bool"(reference=w363, "Colors [4]"=w362) -> ()  [unwired: 1 in, 2 out]
                n269 = property class="Clust (strict)"(reference=w365) -> ("Value"=w369:T1)  [unwired: 1 in, 2 out]
                n270 = local write "Position 3"(w361) -> ()
                n271 = local write "Position 2"(w361) -> ()
                n272 = local write "Position 1"(w361) -> ()
                n273 = Bundle By Name(cluster=w369, "Position 3"=w361, "Position 1"=w361, "Position 2"=w361) -> (w368:T1)
                n274 = local write "WaferAlignment"(w368) -> ()
                n275 = call "StatusGood.vi"("Text.Text"="Please set position 1" ("Status")) -> ()  [unwired: 11 in]
              }
            }
          }
          event "Align Position 2": Value Change {
            # "Set Align to Position 2"
            n276 = event-data() -> ()  [unwired: 1 in, 6 out]
            n277 = case shown="True" "Align Position 2" {
              tunnel: w371 -> [_ w376]
              frame False {
              }
              frame True {
                n278 = Unbundle By Name(w376) -> ("Microsites"=w380:refnum<k24>)
                n279 = call "VXM_MotorPositionF.vi"() -> ("Position"=w377:i32[])  [unwired: 11 in]
                "Position 2" <- w377
                n280 = local read "Steps Per micron"() -> (w383:dbl)
                n281 = local read "Chip Orientation"() -> (w382:i32)
                n282 = control-ref of="Align Position 2"() -> (w384:refnum<vi>)
                n283 = local read "Position 1"() -> (w385:i32[])
                n284 = call "AlignPosition2.vi"("Chip Orientation"=w382, "Steps Per micron"=w383, "Position 1"=w385, "Microsites"=w380, "Boolean in"=w384) -> ("Array"=w373:dbl[], "Numeric"=w374:dbl)  [unwired: 5 in]
                n285 = Unbundle By Name(w376) -> ("ControlRefs.WaferAlignment"=w379:refnum<vi>)
                n286 = local write "Scale Misalign"(w374) -> ()
                n287 = local write "Rotation Misalign"(w373) -> ()
                n288 = property class="Clust (strict)"(reference=w379) -> ("Value"=w378:T1)  [unwired: 1 in, 2 out]
                n289 = Bundle By Name(cluster=w378, "Position 2"=w377, "Scale Misalign"=w374, "Rotation Misalign"=w373) -> (w375:T1)
                n290 = call "StatusGood.vi"("Text.Text"="Please return to position 1 and run cycle" ("Status")) -> ()  [unwired: 11 in]
                n291 = local write "WaferAlignment"(w375) -> ()
              }
            }
          }
        }
        "UiDefinition 3" <- w182
      }
    }
    frame #6 {
      # "Close all tools"
      n292 = local read "VISA resource name"() -> (w387:refnum<visa-resource-name>)
      n293 = flat-sequence {
        frame #0 {
          n294 = call "Vxmdriverlv8.Vi"("Chars to send"="Q") -> ()  [unwired: 21 in, 6 out]
        }
        frame #1 {
          n295 = call "Vxmdriverlv8.Vi"("Close Port"=TRUE) -> ()  [unwired: 21 in, 6 out]
        }
      }
      n296 = call "Close.vi"("VISA resource name"=w387) -> ("error out"=w388:errorcluster)  [unwired: 10 in]
      n297 = call <vilib>:"Simple Error Handler.vi"("error in (no error)"=w388) -> ()  [unwired: 4 in, 5 out]
    }
  }
  n298 = case shown="True" w1 {
    frame False {
    }
    frame True {
      n299 = Stop(stop? (T)=TRUE) -> ()
    }
  }
